vi "GPIO In.vi"() -> ()   [LabVIEW 2020, in "CTI-Scratchpad.lvlib"]
uses:
  CTI-Scratchpad.lvlib
  CTI/GPIO Number.ctl
  CTI/GPIO Direction.ctl
  CTI/Session/Session.lvclass
  CTI/CTI.lvlib
  CTI/VisaComms/VisaComms.lvclass
panel:
  in  "GPIO":T1=16
  in  "Port":refnum<visa-resource-name>="TCPIP::10.190.177.58::5555::SOCKET"
  out "Readback":bool
  in  "stop":bool
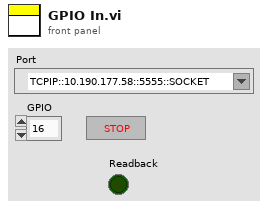
[diagram p1: front panel]
types:
  T1 = typedef "CTI.lvlib/GPIO Number.ctl" = i8
  T2 = typedef "CTI.lvlib/GPIO Direction.ctl" = enum16{"In", "Out"}
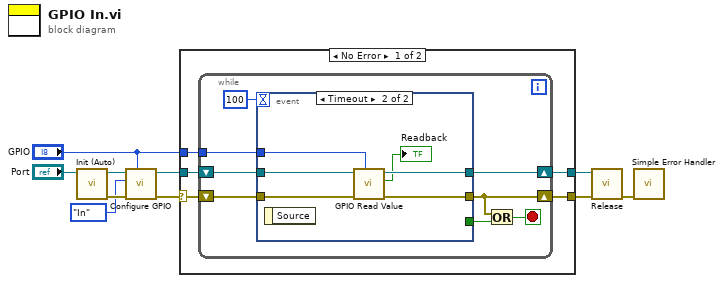
[diagram p0: block diagram]
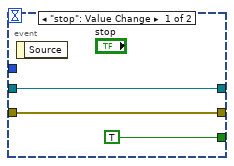
[diagram p2: hidden frame]
diagram:
  n1 = call "Init (Auto).vi"("VISA resource name"="Port") -> ("error out"=w8:errorcluster, "Session"=w9:refnum<class "Session.lvclass">)  [unwired: 8 in, 1 out]
  n2 = call "Configure GPIO.vi"("GPIO #"="GPIO", "error in (no error)"=w8, "GPIO Direction"=GPIO_Direction."In", "Session in"=w9) -> ("error out"=w6:errorcluster, "Session out"=w7:refnum<class "Session.lvclass">)  [unwired: 6 in]
  n3 = case shown="No Error" w6 {
    selector: w6 -> [w14 w33]
    tunnel: w7 -> [w15 w34]
    tunnel: [w13 w34] -> w2
    tunnel: [w12 w33] -> w5
    tunnel: "GPIO" -> [w11 _]
    frame No Error {
      n4 = while {
        shift-right: [w21] -> w13
        shift-left: w15 -> [w23]
        shift-right: [w20] -> w12
        shift-left: w14 -> [w22]
        tunnel: w11 -> [w17]
        stop <- w19 stop-if-true
        n5 = event shown="[1] Timeout" {
          selector: _ -> [_ _]
          dyn-events: _ -> [_ _]
          timeout: 100 -> [_ _]
          tunnel: w23 -> [w26 w28]
          tunnel: w22 -> [w25 w27]
          tunnel: [w26 w32] -> w21
          tunnel: [w25 w31] -> w20
          tunnel: [TRUE _] -> w18
          tunnel: w17 -> [_ w29]
          event "stop": Value Change {
            n6 = event-data() -> ()  [unwired: 1 in, 1 out]
          }
          event Timeout {
            n7 = event-data() -> ()  [unwired: 1 in, 1 out]
            n8 = call "GPIO Read Value.vi"("GPIO #"=w29, "error in (no error)"=w27, "Session in"=w28) -> ("error out"=w31:errorcluster, "Value"=→"Readback":bool, "Session out"=w32:refnum<class "Session.lvclass">)  [unwired: 6 in]
          }
        }
        n9 = Or(x=w20, y=w18) -> (x .or. y?=w19:bool)
      }
    }
    frame Error {
    }
  }
  n10 = call-dynamic "Release.vi"("error in (no error)"=w5, "Session in"=w2) -> ("error out"=w4:errorcluster)  [unwired: 9 in]
  n11 = call <vilib>:"Simple Error Handler.vi"("error in (no error)"=w4) -> ()  [unwired: 4 in, 5 out]
